vi "_Read.vi"(8 "error in (no error)":errorcluster, 11 "Minus in":refnum<class "Minus.lvclass">) -> (0 "error out":errorcluster, 2 "4 Data Points":dbl[](array[numeric]), 3 "Minus out":refnum<class "Minus.lvclass">)   [LabVIEW 2012, in "Minus.lvclass"]
uses:
  Minus.lvclass
  Minus.lvclass/Minus.ctl
  Readable/Readable.lvclass
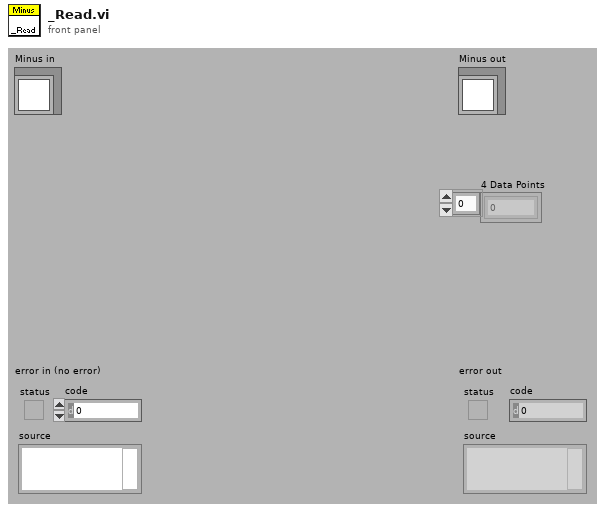
[diagram p1: front panel]
types:
  T1 = typedef "Readable.lvclass/X array.ctl" = T2[]
  T2 = typedef "Readable.lvclass/X.ctl" = dbl
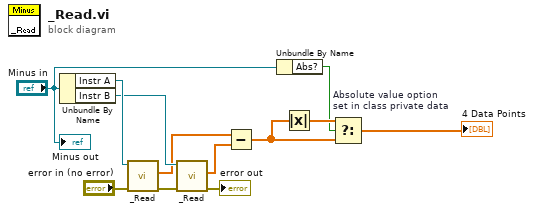
[diagram p0: block diagram]
diagram:
  n1 = Unbundle By Name("Minus in") -> ("Instr A"=w12:refnum<class "Readable.lvclass">, "Instr B"=w11:refnum<class "Readable.lvclass">)
  n2 = call-dynamic "_Read.vi"("error in (no error)"="error in (no error)", "Readable in"=w12) -> ("error out"=w9:errorcluster, "X array"=w7:T1)  [unwired: 8 out]
  n3 = call-dynamic "_Read.vi"("error in (no error)"=w9, "Readable in"=w11) -> ("error out"=→"error out":errorcluster, "X array"=w6:T1)  [unwired: 8 out]
  n4 = Subtract(x=w7, y=w6) -> (x-y=w5:T1)
  n5 = Unbundle By Name("Minus in") -> ("Abs?"=w2:bool)
  n6 = Absolute Value(x=w5) -> (abs(x)=w4:T1)
  n7 = Select "Absolute value option\nset in class private data"(t=w4, s=w2, f=w5) -> (s? t:f=→"4 Data Points":T1)
  "Minus out" <- "Minus in"
